vi "Configure Knock Cylinder Dialog.vi"(5 "Max angle":dbl, 7 "cylinder to be edited":i32, 8 "error in (no error)":errorcluster, 9 "degrees of one u16":dbl, 10 "cylinders in":T1[](array[typedef]), 11 "Item Ref in":T2 format="%.0x") -> (0 "error out":errorcluster, 2 "cylinders out":T1[](array[typedef]), 3 "Item Ref out":T2 format="%.0x")   [LabVIEW 2013, in "Engine Simulation Toolkit System Explorer.lvlib"]
uses:
  Engine Simulation Toolkit System Explorer.lvlib
  Knock Cylinder.ctl
  <vilib>/NI Veristand/Custom Device API/Custom Device Item Ref.ctl
  <vilib>/NI Veristand/Custom Device API/Custom Device API.lvlib
panel:
  in  "Trigger Angle":dbl min=0.0 max=100.0
  in  "Amplitude (V)":dbl=1.0
  in  "Probability (%)":dbl min=0.0 max=100.0 step=0.00152587890625
  in  "Cancel":bool
  in  "OK":bool
  in  "Name":string
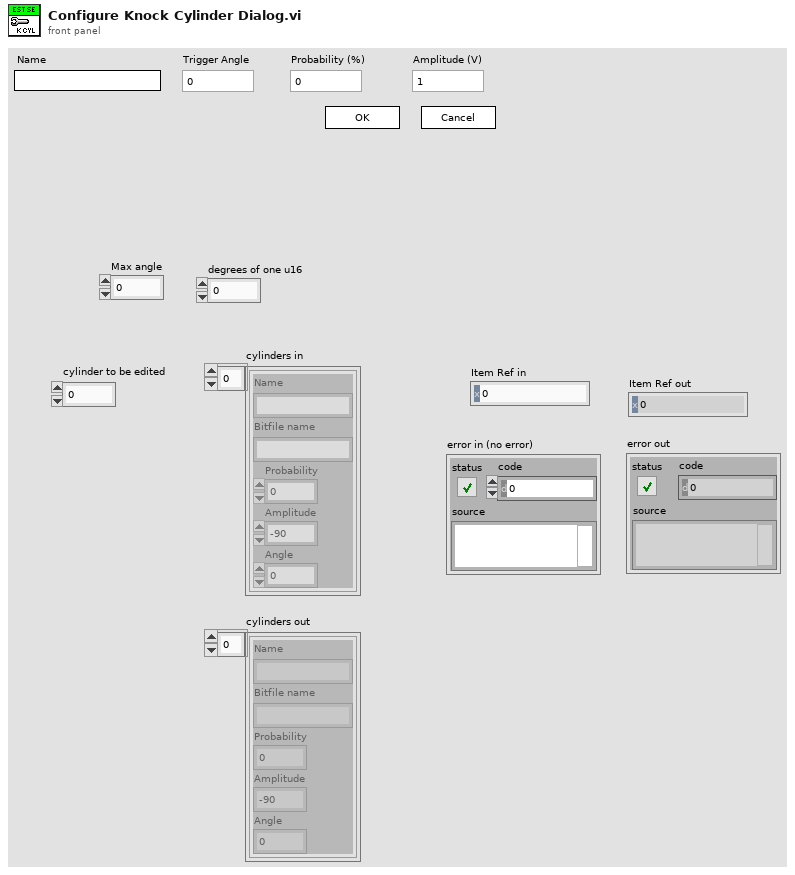
[diagram p1: front panel]
types:
  T1 = typedef "Engine Simulation Toolkit System Explorer.lvlib/Knock Cylinder.ctl" = cluster{"Name":string, "Bitfile name":string, "Probability":dbl, "Amplitude":dbl, "Angle":dbl}
  T2 = typedef "Custom Device API.lvlib/Custom Device Item Ref.ctl" = u64
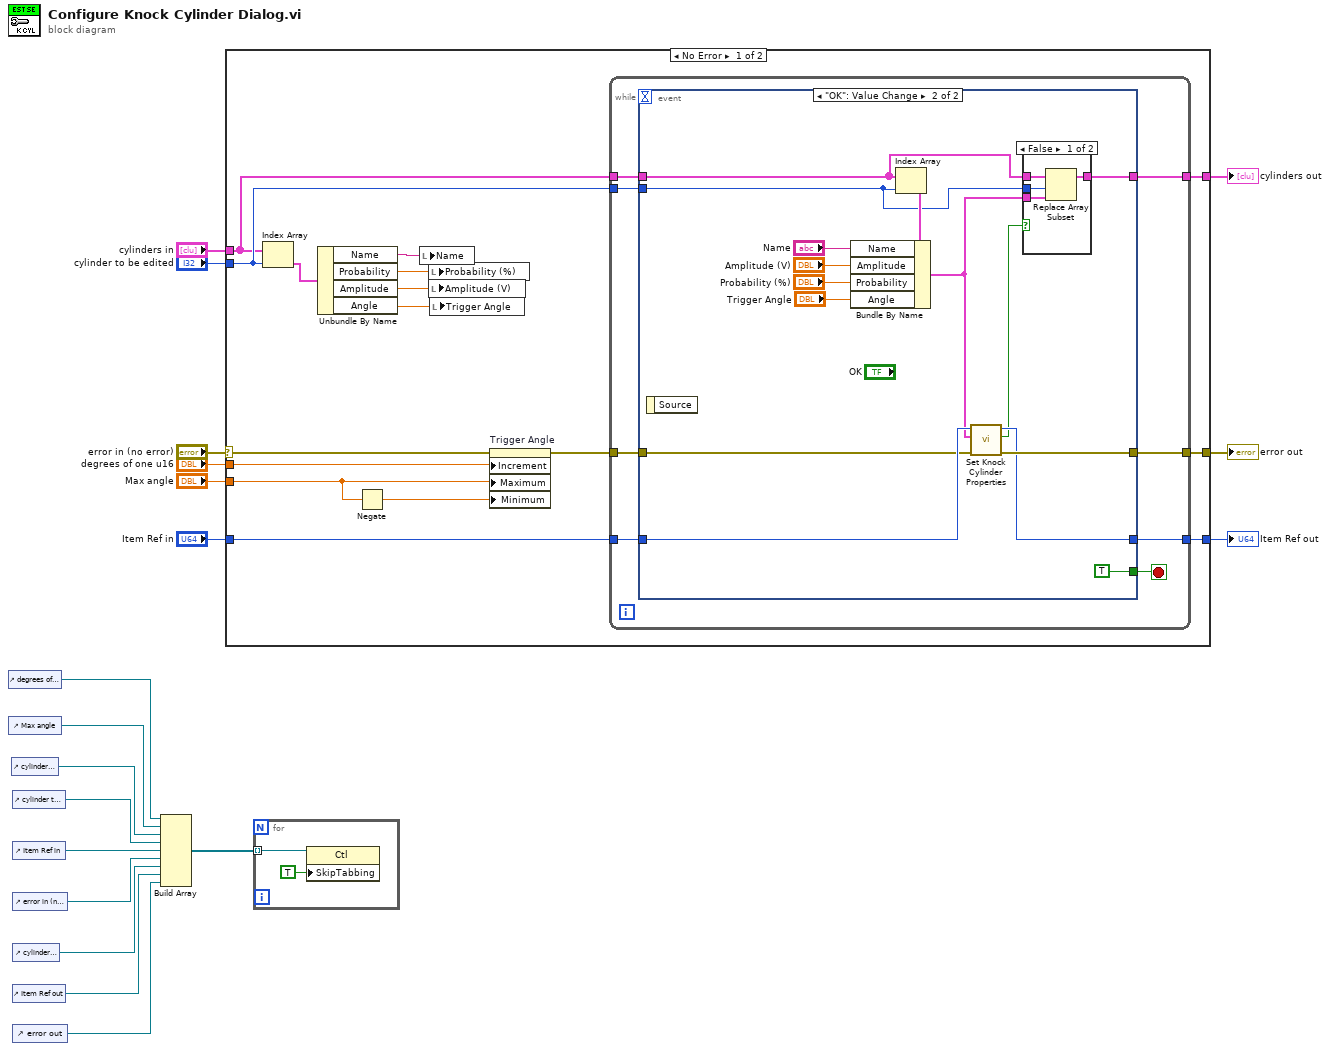
[diagram p0: block diagram]
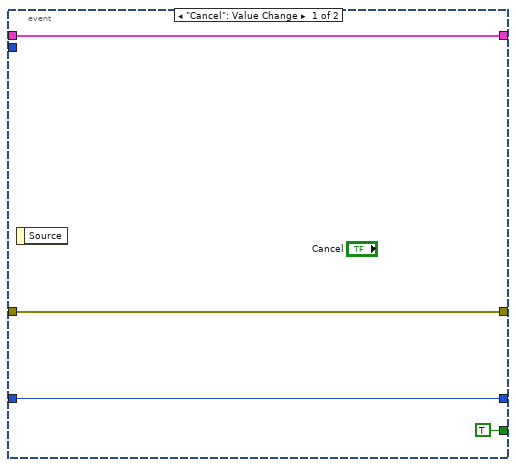
[diagram p2: hidden frame]
diagram:
  n1 = control-ref of="degrees of one u16"() -> (w3:refnum<vi>)
  n2 = control-ref of="Max angle"() -> (w4:refnum<vi>)
  n3 = control-ref of="cylinders out"() -> (w7:refnum<vi>)
  n4 = control-ref of="cylinder to be edited"() -> (w13:refnum<vi>)
  n5 = control-ref of="Item Ref in"() -> (w12:refnum<vi>)
  n6 = control-ref of="error in (no error)"() -> (w11:refnum<vi>)
  n7 = control-ref of="cylinders in"() -> (w10:refnum<vi>)
  n8 = control-ref of="Item Ref out"() -> (w6:refnum<vi>)
  n9 = control-ref of="error out"() -> (w5:refnum<vi>)
  n10 = Build Array(w3, w4, w7, w13, w12, w11, w10, w6, w5) -> (w9:refnum<vi>[])
  n11 = case shown="No Error" "error in (no error)" {
    selector: "error in (no error)" -> [w25 w70]
    tunnel: "cylinders in" -> [w33 w69]
    tunnel: "cylinder to be edited" -> [w34 _]
    tunnel: [w35 w70] -> w16
    tunnel: [w32 w69] -> w8
    tunnel: "Item Ref in" -> [w31 w68]
    tunnel: [w30 w68] -> w14
    tunnel: "degrees of one u16" -> [w23 _]
    tunnel: "Max angle" -> [w21 _]
    frame No Error {
      n12 = Index Array(array=w33, index=w34) -> (element=w28:T1)
      n13 = Unbundle By Name(w28) -> ("Name"=w29:string, "Probability"=w27:dbl, "Amplitude"=w26:dbl, "Angle"=w20:dbl)
      n14 = Negate(x=w21) -> (-x=w22:dbl)
      n15 = local write "Name"(w29) -> ()
      n16 = local write "Probability (%)"(w27) -> ()
      n17 = local write "Amplitude (V)"(w26) -> ()
      n18 = local write "Trigger Angle"(w20) -> ()
      n19 = property on="Trigger Angle" class="DigNum (strict)"(error in=w25, "Increment"=w23, "Maximum"=w21, "Minimum"=w22) -> (error out=w24:errorcluster)  [unwired: 1 in, 1 out]
      n20 = while {
        tunnel: [w36] -> w35
        tunnel: w24 -> [w43]
        tunnel: w34 -> [w42]
        tunnel: w31 -> [w39]
        tunnel: [w38] -> w30
        tunnel: w33 -> [w41]
        tunnel: [w40] -> w32
        stop <- w37 stop-if-true
        n21 = event shown="[1] \"OK\": Value Change" {
          selector: _ -> [_ _]
          dyn-events: _ -> [_ _]
          timeout: _ -> [_ _]
          tunnel: [w47 w57] -> w36
          tunnel: w43 -> [w47 w53]
          tunnel: w42 -> [_ w59]
          tunnel: w41 -> [w46 w60]
          tunnel: [w46 w58] -> w40
          tunnel: w39 -> [w45 w56]
          tunnel: [w45 w55] -> w38
          tunnel: [TRUE TRUE] -> w37
          event "Cancel": Value Change {
            n22 = event-data() -> ()  [unwired: 1 in, 1 out]
          }
          event "OK": Value Change {
            n23 = event-data() -> ()  [unwired: 1 in, 1 out]
            n24 = Index Array(array=w60, index=w59) -> (element=w61:T1)
            n25 = Bundle By Name(cluster=w61, "Name"="Name", "Amplitude"="Amplitude (V)", "Probability"="Probability (%)", "Angle"="Trigger Angle") -> (w49:T1)
            n26 = call "Set Knock Cylinder Properties.vi"("error in (no error)"=w53, "cylinder"=w49, "Item Ref in"=w56) -> ("error out"=w57:errorcluster, "failed"=w54:bool, "Item Ref out"=w55:T2)  [unwired: 6 in]
            n27 = case shown="False" w54 {
              tunnel: w60 -> [w66 w67]
              tunnel: w59 -> [w65 _]
              tunnel: [w64 w67] -> w58
              tunnel: w49 -> [w63 _]
              frame False {
                n28 = Replace Array Subset(array=w66, new element=w63, index=w65) -> (w64:T1[])
              }
              frame True {
              }
            }
          }
        }
      }
    }
    frame Error {
    }
  }
  "error out" <- w16
  "Item Ref out" <- w14
  "cylinders out" <- w8
  n29 = for {
    tunnel: w9 -> [w72] mode=indexing
    n30 = property class="Ctl"(reference=w72, "SkipTabbing"=TRUE ("Skip When Tabbing")) -> ()  [unwired: 1 in, 2 out]
  }
